vi "TCP.IP Server for Ripple Detection - Experiment.vi"() -> ()   [LabVIEW 2021]
doc: "Demonstrates how to set up a basic TCP connection, send data to the specified port once a connection has been established, and terminate the connection once the data has been sent. This VI is designed to stop if the TCP connection is terminated. The data sent in this example is an array of random numbers."
panel:
  out "Elapsed time":dbl format="%.2f"
  out "Waveform Chart":dbl[][](graph)
  out "Iteration terminal":i32
  in  "Stop 2":bool
  in  "File Path":path
  in  "Number of row to read \nat a time":i32=10000
  out "Waveform Graph 10":dbl[](graph)
  in  "loop 1":i32
  in  "Client Closed":string="The client VI closed the connection."
  in  "Stop":bool
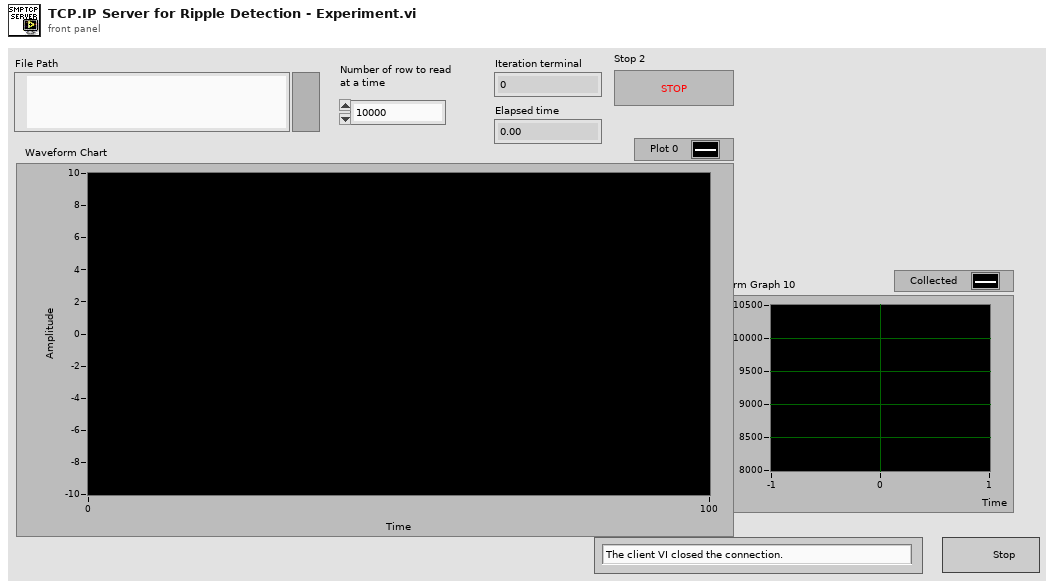
[diagram p1: front panel]
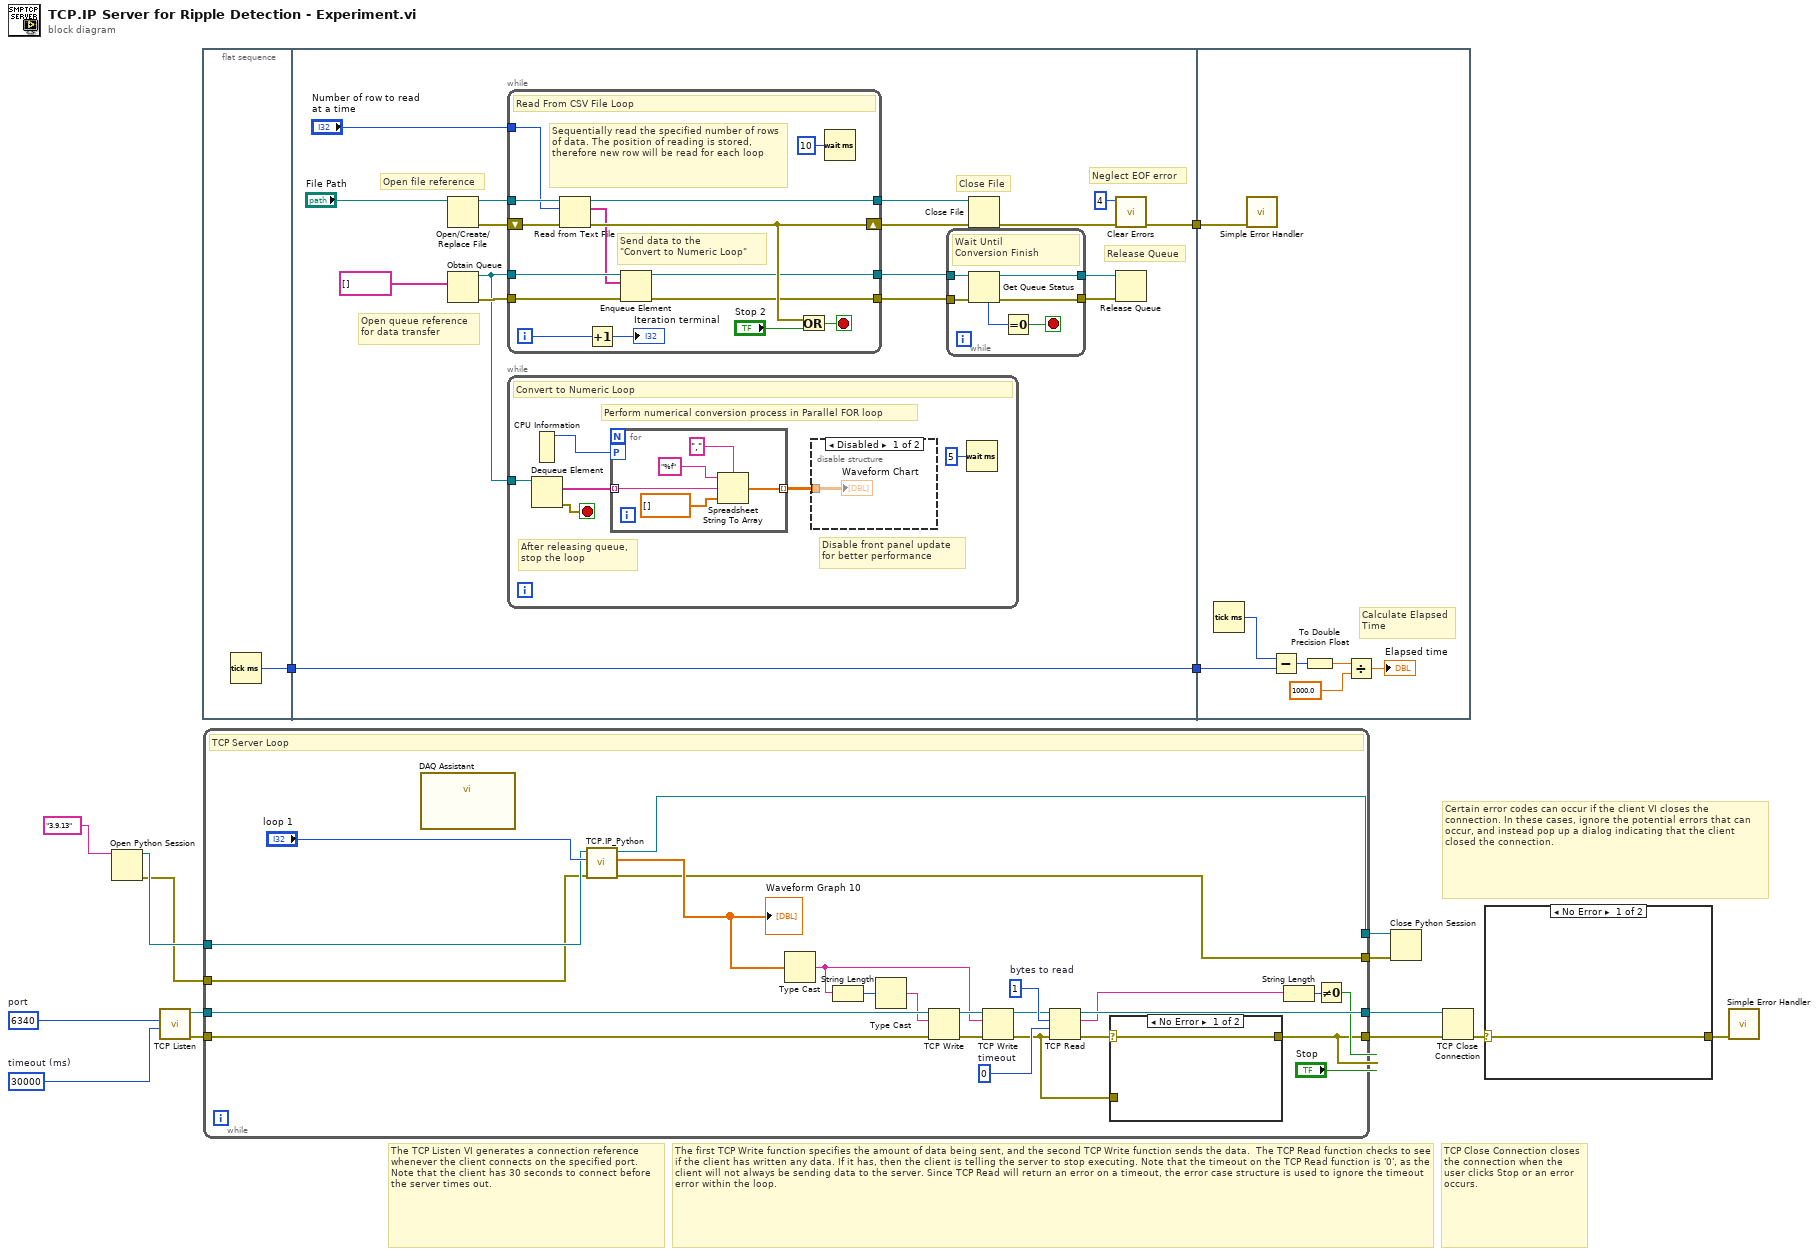
[diagram p0: block diagram]
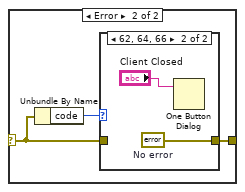
[diagram p3: hidden frame]
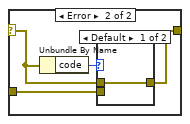
[diagram p5: hidden frame]
diagram:
  w9 = u16 6340  # port
  w10 = 30000  # timeout (ms)
  # "TCP Close Connection closes the connection when the user clicks Stop or an error occurs."
  # "The TCP Listen VI generates a connection reference whenever the client connects on the specified port. Note that the client has 30 seconds to connect before the server times out."
  # "Certain error codes can occur if the client VI closes the connection. In these cases, ignore the potential errors that can occur, and instead pop up a dialog indicating that the client closed the connection."
  # "The first TCP Write function specifies the amount of data being sent, and the second TCP Write function sends the data.  The TCP Read function checks to see if the client has written any data. If it has, then the client is telling the server to stop executing. Note that the timeout on the TCP Read function is '0', as the client will not always be sending data to the server. Since TCP Read will return an error on a timeout, the error case structure is used to ignore the timeout error within the loop."
  n1 = Open Python Session(python version="3.9.13" ("Python version")) -> (session out=w7:refnum<k35>, error out=w6:errorcluster)  [unwired: 2 in]
  n2 = call <vilib>:"TCP Listen.vi"("timeout ms (wait forever: -1)"=w10, "port"=w9) -> ("error out"=w11:errorcluster, "connection ID"=w12:refnum<k5>)  [unwired: 5 in, 3 out]
  n3 = flat-sequence {
    tunnel: [w17] -> w3
    tunnel: w3 -> [w29]
    tunnel: [w29] -> w2
    tunnel: [w27] -> w1
    tunnel: w2 -> [w73]
    tunnel: w1 -> [w72]
    frame #0 {
      n4 = Tick Count (ms)() -> (millisecond timer value=w17:u32)
    }
    frame #1 {
      # "Neglect EOF error"
      # "Release Queue"
      # "Close File"
      # "Open queue reference\nfor data transfer"
      # "Open file reference"
      n5 = Open/Create/Replace File(file path (use dialog)="File Path") -> (refnum out=w34:refnum<file>, error out=w33:errorcluster)  [unwired: 5 in, 1 out]
      n6 = Obtain Queue(element data type=string[] [] ("形式文字列")) -> (queue out=w22:refnum<queue>, error out=w23:errorcluster)  [unwired: 4 in, 1 out]
      n7 = while {
        tunnel: w34 -> [w55]
        tunnel: [w53] -> w31
        shift-right: [w48] -> w30
        shift-left: w33 -> [w54]
        tunnel: "Number of row to read \nat a time" -> [w49]
        tunnel: w22 -> [w47]
        tunnel: w23 -> [w46]
        tunnel: [w44] -> w21
        tunnel: [w43] -> w20
        i -> [w51]
        stop <- w52 stop-if-true
        # "Send data to the \n\"Convert to Numeric Loop\""
        # "Sequentially read the specified number of rows of data. The position of reading is stored, therefore new row will be read for each loop"
        # "Read From CSV File Loop"
        n8 = Read from Text File(file (use dialog)=w55, count=w49, error in=w54) -> (refnum out=w53:refnum<file>, text=w45:string[], error out=w48:errorcluster)  [unwired: 1 in, 1 out]
        n9 = Increment(x=w51) -> (x+1=→"Iteration terminal":i32)
        n10 = Enqueue Element(queue=w47, element=w45, error in (no error)=w46) -> (queue out=w44:refnum<queue>, error out=w43:errorcluster)  [unwired: 1 in, 1 out]
        n11 = Or(x=w48, y="Stop 2") -> (x .or. y?=w52:bool)
        n12 = Wait (ms)(milliseconds to wait=u32 10 ("ミリ秒待機時間")) -> ()  [unwired: 1 out]
      }
      n13 = while {
        tunnel: w22 -> [w61]
        stop <- w58 stop-if-true
        # "Disable front panel update \nfor better performance"
        # "After releasing queue,\nstop the loop"
        # "Perform numerical conversion process in Parallel FOR loop"
        # "Convert to Numeric Loop"
        n14 = CPU Information() -> (4:w57:i32)  [unwired: 3 out]
        n15 = Dequeue Element(queue=w61) -> (element=w60:string[], error out=w58:errorcluster)  [unwired: 2 in, 2 out]
        n16 = for "Forループ" {
          tunnel: w60 -> [w64] mode=indexing
          tunnel: [w65] -> w59 mode=indexing
          workers-P: w57 -> [_]
          n17 = Spreadsheet String To Array(delimiter (Tab)="," ("デリミタ（タブ）"), format string="%f" ("形式文字列"), spreadsheet string=w64, array type (2D Dbl)=dbl[] []) -> (array=w65:dbl[])
        }
        n18 = disable-structure shown="Disabled" {
          disable-tunnel: w59 -> [w62 _]
          frame Disabled {
            "Waveform Chart" <- w62
          }
          frame Enabled {
          }
        }
        n19 = Wait (ms)(milliseconds to wait=u32 5 ("ミリ秒待機時間")) -> ()  [unwired: 1 out]
      }
      n20 = while {
        tunnel: w21 -> [w40]
        tunnel: w20 -> [w39]
        tunnel: [w36] -> w18
        tunnel: [w35] -> w19
        stop <- w37 stop-if-true
        # "Wait Until \nConversion Finish"
        n21 = Get Queue Status(queue=w40, error in (no error)=w39) -> (queue out=w36:refnum<queue>, error out=w35:errorcluster, # elements in queue=w38:i32)  [unwired: 1 in, 5 out]
        n22 = Equal To 0?(x=w38) -> (x = 0?=w37:bool)
      }
      n23 = Close File(refnum=w31, error in=w30) -> (error out=w28:errorcluster)  [unwired: 1 out]
      n24 = call <vilib>:"Clear Errors.vi"("error in (no error)"=w28, "specific error code to clear (0: all)"=4) -> ("error out"=w27:errorcluster)  [unwired: 4 in, 1 out]
      n25 = Release Queue(queue=w18, error in (no error)=w19) -> ()  [unwired: 1 in, 3 out]
    }
    frame #2 {
      # "Calculate Elapsed\nTime"
      n26 = Tick Count (ms)() -> (millisecond timer value=w74:u32)
      n27 = call <vilib>:"Simple Error Handler.vi"("error in (no error)"=w72) -> ()  [unwired: 4 in, 5 out]
      n28 = Subtract(x=w74, y=w73) -> (x-y=w71:u32)
      n29 = To Double Precision Float(number=w71) -> (double precision float=w70:dbl)
      n30 = Divide(x=w70, y=1000.0) -> (x/y=→"Elapsed time":dbl)
    }
  }
  n31 = while {
    tunnel: [w82] -> w15
    tunnel: [w88] -> w16
    tunnel: w12 -> [w99]
    tunnel: w11 -> [w92]
    tunnel: w7 -> [w78]
    tunnel: w6 -> [w77]
    tunnel: [w76] -> w5
    tunnel: [w75] -> w4
    stop <- w93 stop-if-true
    w87 = 0  # timeout
    w90 = 1  # bytes to read
    # "TCP Server Loop"
    n32 = call "DAQ Assistant"() -> ()  [unwired: 12 in]
    n33 = call "TCP.IP_Python.vi"("error in (no error)"=w77, "loop 1"="loop 1", "Refnum in"=w78) -> ("error out"=w75:errorcluster, "Array"=w79:dbl[], "Refnum out"=w76:refnum<k35>)  [unwired: 6 in]
    "Waveform Graph 10" <- w79
    n34 = Type Cast(x=w79) -> (*(type *) &x=w94:string)  [unwired: 1 out]
    n35 = String Length(string=w94) -> (length=w96:i32)
    n36 = Type Cast(x=w96) -> (*(type *) &x=w95:string)  [unwired: 1 out]
    n37 = TCP Write(connection ID=w99, data in=w95, error in (no error)=w92) -> (connection ID out=w98:refnum<k5>, error out=w97:errorcluster)  [unwired: 2 out]
    n38 = TCP Write(connection ID=w98, data in=w94, error in (no error)=w97) -> (connection ID out=w89:refnum<k5>, error out=w81:errorcluster)  [unwired: 2 out]
    n39 = TCP Read(connection ID=w89, bytes to read=w90, error in (no error)=w81, 9:w87) -> (connection ID out=w88:refnum<k5>, data out=w85:string, error out=w83:errorcluster)  [unwired: 1 out]
    n40 = case shown="No Error" w83 {
      selector: w83 -> [w100 w103]
      tunnel: [w100 w101] -> w82
      tunnel: w81 -> [_ w102]
      frame No Error {
      }
      frame Error {
        n41 = Unbundle By Name(w103) -> ("code"=w104:i32)
        n42 = case shown="Default" w104 {
          tunnel: w103 -> [w105 _]
          tunnel: w102 -> [_ w106]
          tunnel: [w105 w106] -> w101
          frame Default {
          }
          frame 56 {
          }
        }
      }
    }
    n43 = String Length(string=w85) -> (length=w86:i32)
    n44 = Not Equal To 0?(x=w86) -> (x != 0?=w84:bool)
    n45 = Compound Arithmetic op=OR(w84, w82, "Stop") -> (w93:bool)
  }
  n46 = Close Python Session(session in=w5, error in=w4) -> ()  [unwired: 1 out]
  n47 = TCP Close Connection(connection ID=w16, error in (no error)=w15) -> (error out=w14:errorcluster)  [unwired: 2 out]
  n48 = case shown="No Error" w14 {
    selector: w14 -> [w107 w109]
    tunnel: [w107 w108] -> w13
    frame No Error {
    }
    frame Error {
      n49 = Unbundle By Name(w109) -> ("code"=w110:i32)
      n50 = case shown="62, 64, 66" w110 {
        tunnel: w109 -> [w111 _]
        tunnel: [w111 w113] -> w108
        frame Default {
        }
        frame 62, 64, 66 {
          w113 = errorcluster {"status"=FALSE, "code"=0, "source"=""}  # No error
          n51 = One Button Dialog(message="Client Closed") -> ()  [unwired: 1 in, 1 out]
        }
      }
    }
  }
  n52 = call <vilib>:"Simple Error Handler.vi"("error in (no error)"=w13) -> ()  [unwired: 1 in, 8 out]
